vi "WriteMaxTimeout.vi"(8 "error in (no error)":errorcluster, 11 "Subsystem in":refnum<class "Subsystem.lvclass">) -> (0 "error out":errorcluster, 3 "Subsystem out":refnum<class "Subsystem.lvclass">)   [LabVIEW 2017, in "Subsystem.lvclass"]
uses:
  Subsystem.lvclass
  Subsystem.lvclass/Subsystem.ctl
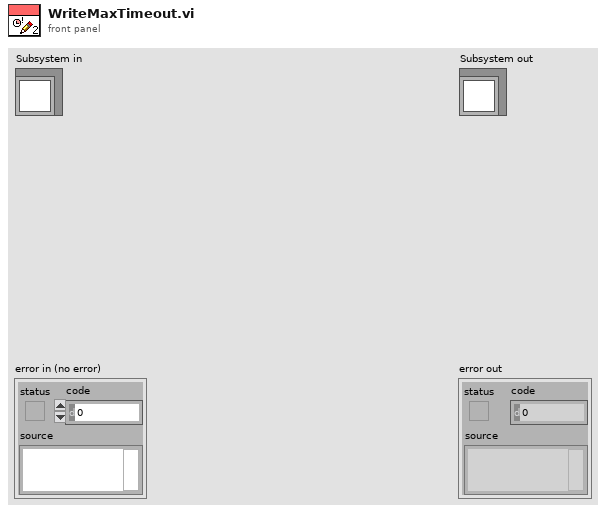
[diagram p1: front panel]
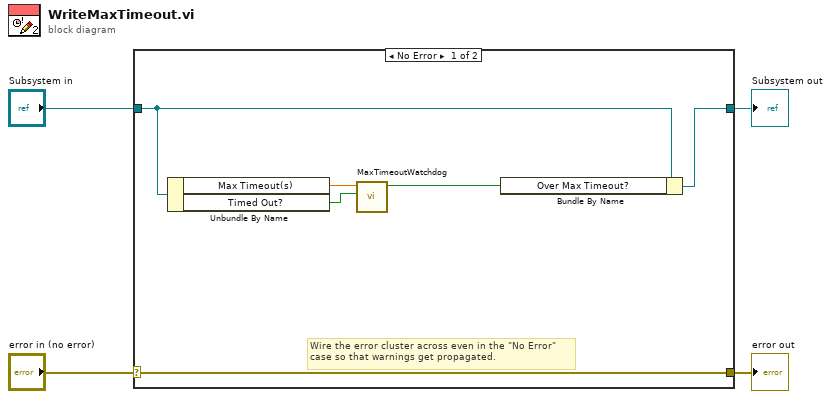
[diagram p0: block diagram]
diagram:
  n1 = case shown="No Error" "error in (no error)" {
    selector: "error in (no error)" -> [w9 w12]
    tunnel: [w9 w12] -> w3
    tunnel: [w6 w11] -> w1
    tunnel: "Subsystem in" -> [w7 w11]
    frame No Error {
      # "Wire the error cluster across even in the \"No Error\"\ncase so that warnings get propagated."
      n2 = Unbundle By Name(w7) -> ("Max Timeout(s)"=w5:dbl, "Timed Out?"=w10:bool)
      n3 = call "MaxTimeoutWatchdog.vi"("Keep counting?"=w10, "Max Timeout (s)"=w5) -> ("Over Max Timeout?"=w8:bool)  [unwired: 9 in]
      n4 = Bundle By Name(cluster=w7, "Over Max Timeout?"=w8) -> (w6:refnum<class "Subsystem.lvclass">)
    }
    frame Error {
    }
  }
  "error out" <- w3
  "Subsystem out" <- w1
